vi "Kinesis - BBD202 - Two Axis Scan.vi"() -> ()   [LabVIEW 2021]
doc: "2D motor scan example Vi."
uses:
  U:/Kinesis LabVIEW Website Examples/Thorlabs.MotionControl.Controls.dll
  U:/Kinesis LabVIEW Website Examples/Thorlabs.MotionControl.Benchtop.BrushlessMotorCLI.dll
panel:
  in  "SerialNumber":string
  in  "milliseconds to wait 3":u32
  in  "Settle Time":u32=5000
  in  "stop":bool
  in  "?":bool
  in  "Y":sgl
  in  "X":sgl
  in  "BenchtopBrushlessControl 2":refnum<k24>(container)
  in  "BenchtopBrushlessControl":refnum<k24>(container)
  in  "Num Of Steps":i32=4
  in  "Step Size (mm)":sgl=0.25 format="%.2f"
  # "Notes:"
  # "- Ensure that the appropriate .DLLs are copied into your Project Folder. Check that the correct bit type are used depending on your version of LabVIEW\ni.e. 32-bit or 64-bit.\n\n\n\n\n\n\n\n\n\n\n\n\n\n\n- Open the example VI through the LabVIEW Project Explorer to correctly load the User Interface from Thorlabs.MotionControl.Controls.dll."
  # "Thorlabs Hardware: BBD202 Benchtop Stepper Motor Controller\nhttps://www.thorlabs.com/newgrouppage9.cfm?objectgroup_id=5066\n\nDescription: This VI will enable you to connect to a BBD202 controller. The VI will perform a 2D square raster scan, moving in a forward direction from a user defined start position. You will be able to set the number of steps, step size, as well as the settle time - how long the stage settles at a scanned position.\n\nInstructions: \n1) Connect your BBD202 to your PC & power the device. For full device setup, the device product manual can be found on our website here. - https://www.thorlabs.com/thorproduct.cfm?partnumber=BBD202\n3) Enter the device serial number below.\n4) Click 'Run' in the LabVIEW Toolbar.\n5) After running the VI, edit the Scan Parameters: Step Size, Number of Steps (X & Y), milliseconds to wait.\n6) To start the scan click 'START SCAN'.\n7) To end the VI click 'END' to safely disconnect the device."
  # "Example Image of .NET Controller - VI opened via Project Explorer/ not opened via Project Explorer"
  # "VI Not Opened via Project Explorer"
  # "VI Opened via Project Explorer"
  # "Start Position"
  # "- To explore the range of methods available, please visit the .NET API, included with your Kinesis software.\n\n- For tips on building your own VIs with Thorlabs Motion Control Hardware, please see our LabVIEW Guide here.\nhttps://www.thorlabs.com/newgrouppage9.cfm?objectgroup_id=10285"
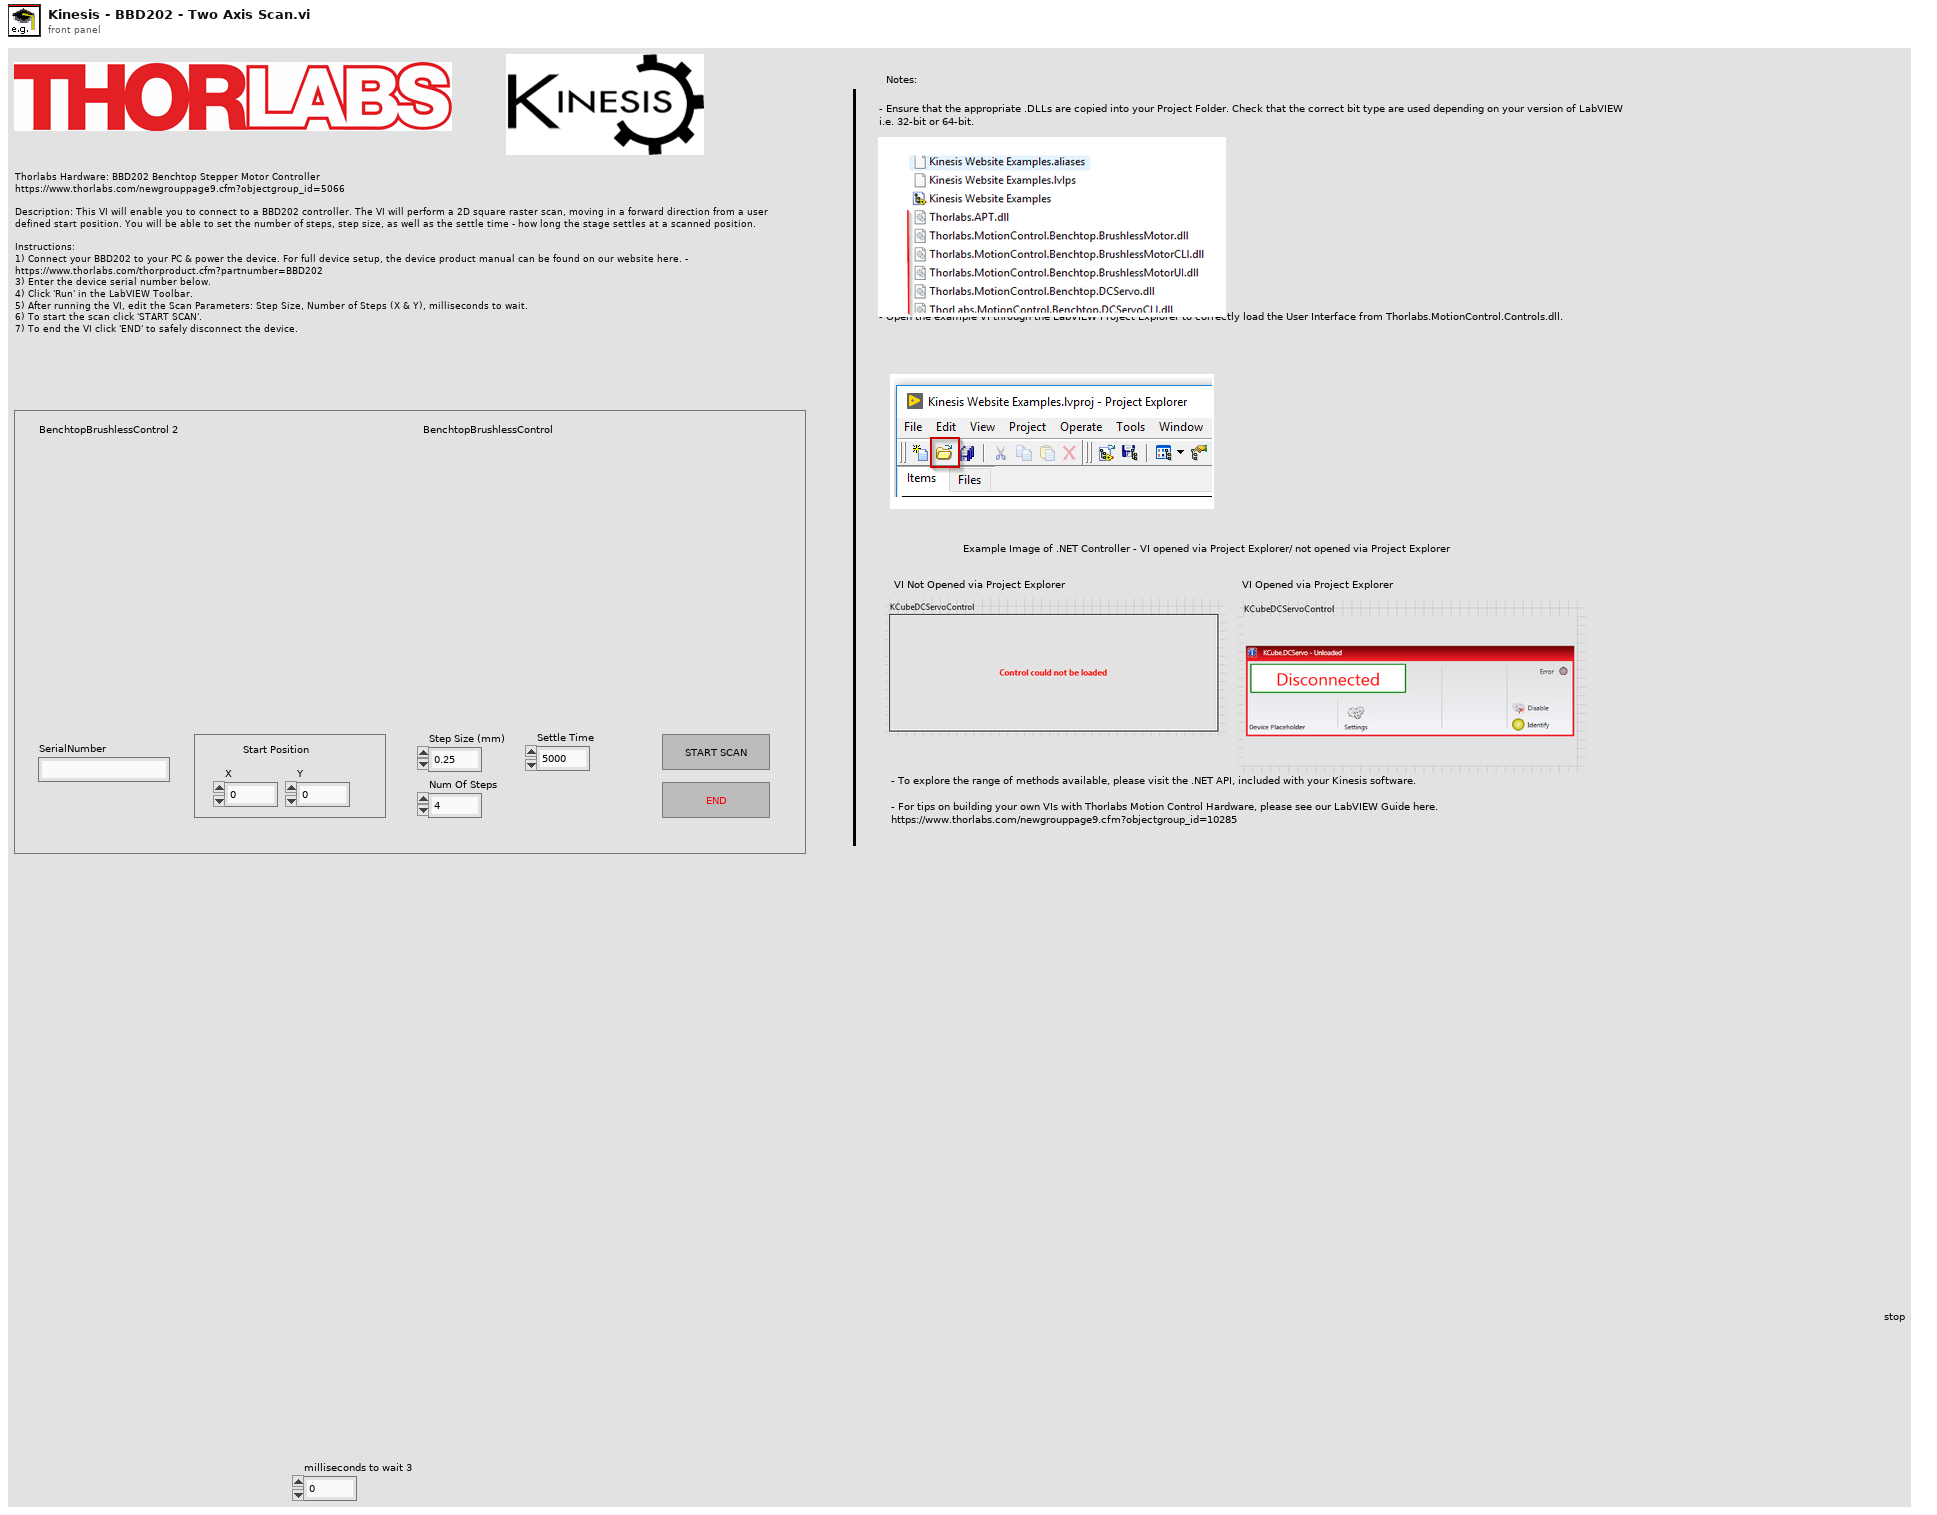
[diagram p1: front panel]
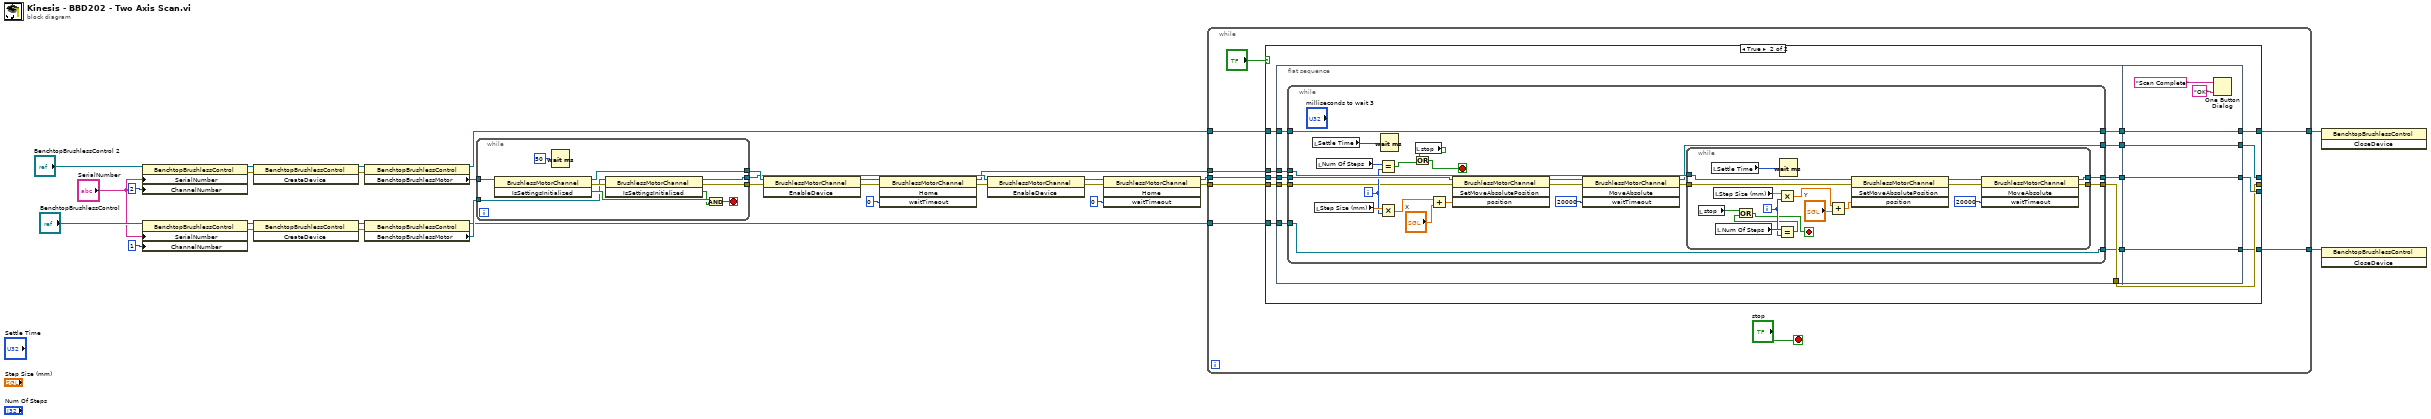
[diagram p0: block diagram]
diagram:
  n1 = property class="BenchtopBrushlessControl"(reference="BenchtopBrushlessControl 2", "SerialNumber"="SerialNumber", "ChannelNumber"=2) -> (reference out=w27:refnum<k24>, error out=w18:errorcluster)  [unwired: 1 in]
  n2 = property class="BenchtopBrushlessControl"(reference="BenchtopBrushlessControl", "SerialNumber"="SerialNumber", "ChannelNumber"=1) -> (reference out=w31:refnum<k24>, error out=w17:errorcluster)  [unwired: 1 in]
  n3 = invoke class="BenchtopBrushlessControl" method="CreateDevice"(reference=w27, error in=w18) -> (reference out=w26:refnum<k24>, error out=w16:errorcluster)  [unwired: 1 in, 1 out]
  n4 = invoke class="BenchtopBrushlessControl" method="CreateDevice"(reference=w31, error in=w17) -> (reference out=w30:refnum<k24>, error out=w15:errorcluster)  [unwired: 1 in, 1 out]
  n5 = property class="BenchtopBrushlessControl"(reference=w26, error in=w16) -> (reference out=w4:refnum<k24>, "BenchtopBrushlessMotor"=w6:refnum<k24>)  [unwired: 1 out]
  n6 = property class="BenchtopBrushlessControl"(reference=w30, error in=w15) -> (reference out=w5:refnum<k24>, "BenchtopBrushlessMotor"=w7:refnum<k24>)  [unwired: 1 out]
  n7 = while {
    tunnel: [w39] -> w20
    tunnel: [w38] -> w19
    tunnel: [w36] -> w9
    tunnel: w7 -> [w34]
    tunnel: w6 -> [w33]
    stop <- w40 stop-if-true
    n8 = invoke class="BrushlessMotorChannel" method="IsSettingsInitialized"(reference=w33) -> (reference out=w39:refnum<k24>, error out=w35:errorcluster, "IsSettingsInitialized"=w42:bool)  [unwired: 2 in]
    n9 = Wait (ms)(milliseconds to wait=u32 50) -> ()  [unwired: 1 out]
    n10 = invoke class="BrushlessMotorChannel" method="IsSettingsInitialized"(reference=w34, error in=w35) -> (reference out=w38:refnum<k24>, error out=w36:errorcluster, "IsSettingsInitialized"=w41:bool)  [unwired: 1 in]
    n11 = And(x=w42, y=w41) -> (x .and. y?=w40:bool)
  }
  n12 = invoke class="BrushlessMotorChannel" method="EnableDevice"(reference=w20, error in=w9) -> (reference out=w22:refnum<k24>, error out=w14:errorcluster)  [unwired: 1 in, 1 out]
  n13 = invoke class="BrushlessMotorChannel" method="Home"(reference=w22, error in=w14, "waitTimeout"=0) -> (reference out=w10:refnum<k24>, error out=w8:errorcluster)  [unwired: 1 in, 2 out]
  n14 = invoke class="BrushlessMotorChannel" method="EnableDevice"(reference=w19, error in=w8) -> (reference out=w21:refnum<k24>, error out=w13:errorcluster)  [unwired: 1 in, 1 out]
  n15 = invoke class="BrushlessMotorChannel" method="Home"(reference=w21, error in=w13, "waitTimeout"=0) -> (reference out=w11:refnum<k24>, error out=w12:errorcluster)  [unwired: 1 in, 2 out]
  n16 = while {
    tunnel: w11 -> [w51]
    tunnel: w12 -> [w48]
    tunnel: w10 -> [w50]
    tunnel: w5 -> [w47]
    tunnel: w4 -> [w46]
    tunnel: [w45] -> w3
    tunnel: [w44] -> w2
    stop <- "stop" stop-if-true
    n17 = case shown="True" "?" {
      tunnel: [w56 w70] -> _
      tunnel: [w55 w69] -> _
      tunnel: w50 -> [w55 w68]
      tunnel: w51 -> [w56 w67]
      tunnel: w48 -> [w54 w64]
      tunnel: [w54 w63] -> _
      tunnel: w47 -> [w53 w62]
      tunnel: w46 -> [w52 w61]
      tunnel: [w53 w60] -> w45
      tunnel: [w52 w58] -> w44
      frame False {
      }
      frame True {
        n18 = flat-sequence {
          tunnel: w68 -> [w78]
          tunnel: w67 -> [w77]
          tunnel: [w80] -> w66
          tunnel: [w79] -> w65
          tunnel: w64 -> [w76]
          tunnel: [w75] -> w63
          tunnel: w62 -> [w74]
          tunnel: w61 -> [w73]
          tunnel: [w72] -> w59
          tunnel: [w71] -> w57
          tunnel: [w124] -> w69
          tunnel: [w125] -> w70
          tunnel: w66 -> [w125]
          tunnel: w65 -> [w124]
          tunnel: [w121] -> w60
          tunnel: w59 -> [w121]
          tunnel: [w120] -> w58
          tunnel: w57 -> [w120]
          frame #0 {
            n19 = while {
              tunnel: w77 -> [w99]
              tunnel: w78 -> [w98]
              tunnel: [w96] -> w80
              tunnel: [w95] -> w79
              tunnel: w76 -> [w88]
              tunnel: [w86] -> w75
              tunnel: [w85] -> w72
              tunnel: w74 -> [w85]
              tunnel: [w84] -> w71
              tunnel: w73 -> [w84]
              i -> [w89]
              stop <- w82 stop-if-true
              n20 = local read "Settle Time"() -> (w90:u32)
              n21 = local read "Step Size (mm)"() -> (w102:sgl)
              n22 = local read "Num Of Steps"() -> (w101:i32)
              n23 = Equal?(x=w101, y=w89) -> (x = y?=w83:bool)
              n24 = Multiply(x=w102, y=w89) -> (x*y=w93:sgl)
              n25 = Wait (ms)(milliseconds to wait=w90) -> ()  [unwired: 1 out]
              n26 = local read "stop"() -> (w81:bool)
              n27 = Or(x=w81, y=w83) -> (x .or. y?=w82:bool)
              n28 = Add(x=w93, y="X") -> (x+y=w92:sgl)
              n29 = invoke class="BrushlessMotorChannel" method="SetMoveAbsolutePosition"(reference=w99, error in=w88, "position"=w92) -> (reference out=w100:refnum<k24>, error out=w94:errorcluster)  [unwired: 1 in, 2 out]
              n30 = invoke class="BrushlessMotorChannel" method="MoveAbsolute"(reference=w100, error in=w94, "waitTimeout"=20000) -> (reference out=w96:refnum<k24>, error out=w87:errorcluster)  [unwired: 1 in, 2 out]
              n31 = while {
                tunnel: w98 -> [w116]
                tunnel: [w114] -> w95
                tunnel: w87 -> [w113]
                tunnel: [w111] -> w86
                i -> [w106]
                stop <- w104 stop-if-true
                n32 = local read "stop"() -> (w103:bool)
                n33 = local read "Settle Time"() -> (w107:u32)
                n34 = local read "Step Size (mm)"() -> (w119:sgl)
                n35 = local read "Num Of Steps"() -> (w118:i32)
                n36 = Multiply(x=w119, y=w106) -> (x*y=w110:sgl)
                n37 = Equal?(x=w118, y=w106) -> (x = y?=w105:bool)
                n38 = Or(x=w103, y=w105) -> (x .or. y?=w104:bool)
                n39 = Wait (ms)(milliseconds to wait=w107) -> ()  [unwired: 1 out]
                n40 = Add(x=w110, y="Y") -> (x+y=w109:sgl)
                n41 = invoke class="BrushlessMotorChannel" method="SetMoveAbsolutePosition"(reference=w116, error in=w113, "position"=w109) -> (reference out=w117:refnum<k24>, error out=w112:errorcluster)  [unwired: 1 in, 2 out]
                n42 = invoke class="BrushlessMotorChannel" method="MoveAbsolute"(reference=w117, error in=w112, "waitTimeout"=20000) -> (reference out=w114:refnum<k24>, error out=w111:errorcluster)  [unwired: 1 in, 2 out]
              }
            }
          }
          frame #1 {
            n43 = One Button Dialog(message="Scan Complete", button name ("OK")="OK") -> ()  [unwired: 1 out]
          }
        }
      }
    }
  }
  n44 = invoke class="BenchtopBrushlessControl" method="CloseDevice"(reference=w2) -> ()  [unwired: 2 in, 3 out]
  n45 = invoke class="BenchtopBrushlessControl" method="CloseDevice"(reference=w3) -> ()  [unwired: 2 in, 3 out]
